vi "Grafica croce.vi"() -> ()   [LabVIEW 2016]
panel:
  out "XY Graph":cluster{"X":dbl[], "Y":dbl[]}(graph)
  in  "TOLL H %":dbl format="%#_13g"
  in  "TOLL Q %":dbl format="%#_13g"
  in  "H":dbl format="%#_13g"
  in  "Q":dbl format="%#_13g"
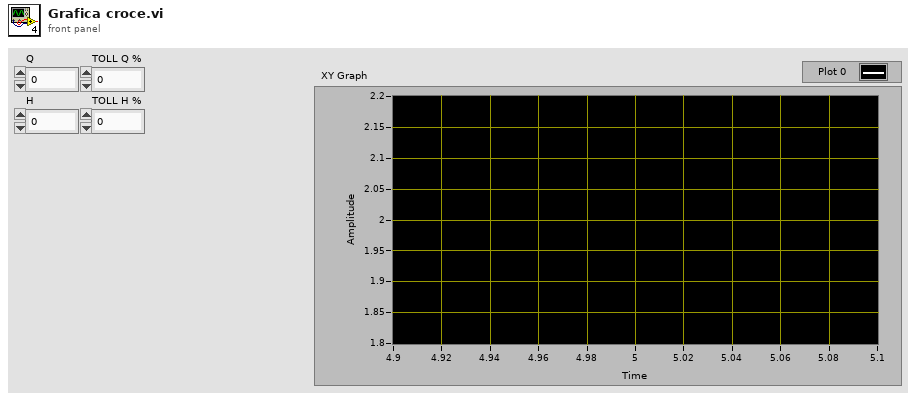
[diagram p1: front panel]
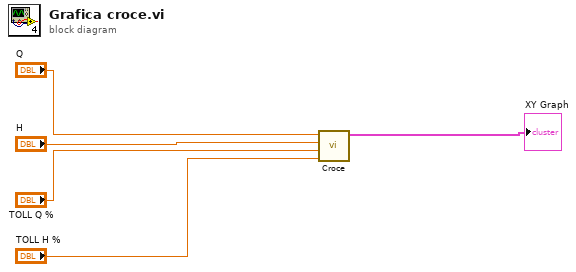
[diagram p0: block diagram]
diagram:
  n1 = call "Croce.vi"("TOLL H %"="TOLL H %", "TOLL Q %"="TOLL Q %", "H"="H", "Q"="Q") -> ("element"=→"XY Graph":cluster{"X":dbl[], "Y":dbl[]})  [unwired: 7 in]
